vi "Start Measurement.vi"(8 "error in (no error)":errorcluster, 10 "Launch Measurements Message in":refnum<class "Launch Measurements Message.lvclass">, 11 "Controller in":refnum<class "Controller.lvclass">) -> (0 "error out":errorcluster, 3 "Controller out":refnum<class "Controller.lvclass">)   [LabVIEW 2016, in "Controller Actor.lvlib" / "Controller.lvclass"]
uses:
  <userlib>/Common Components/Controller/Controller.lvclass
  C:/Program Files (x86)/National Instruments/LabVIEW 2016/vi.lib/ActorFramework/Actor/Actor.lvclass
  <userlib>/Common Components/Controller/Messages/Launch Measurements Message/Launch Measurements Message.lvclass
  <userlib>/Common Components/Controller/Messages/Launch Measurements Message/Launch Measurements Message.lvclass/Launch Measurements Message.ctl
  <userlib>/Common Components/Function Actor/Function.lvclass/Function.ctl
  <vilib>/ActorFramework/Actor/Actor.lvclass/Actor.ctl
  <vilib>/ActorFramework/Message Enqueuer/Message Enqueuer.lvclass/Message Enqueuer.ctl
  <userlib>/Common Components/Function Actor/Accessors/Write Time Measurement Requested.vi
  <userlib>/Common Components/Function Actor/Write GUID.vi
  <userlib>/Common Components/Controller/Messages/Launch Measurements Message/Read Measurement Name.vi
  <userlib>/Common Components/Controller/Messages/Launch Measurements Message/Read Device Names.vi
  <userlib>/Common Components/Controller/Messages/Launch Measurements Message/Read Show FP_.vi
  <userlib>/Common Components/Controller/Messages/Launch Measurements Message/Read Time Measurement Requested 2.vi
  <userlib>/Common Components/Controller/Messages/Launch Measurements Message/Read GUID.vi
  <vilib>/ActorFramework/Message Enqueuer/Init from Existing Queue.vi
  <userlib>/Common Components/Function Actor/Function.lvclass
  <userlib>/Common Components/Function Actor/Properties/Write Array of Hardware 2.vi
  <userlib>/Common Components/Function Actor/Properties/Write Show UI While Running 2.vi
  <vilib>/ActorFramework/Message Enqueuer/Message Enqueuer.lvclass
  <vilib>/ActorFramework/Actor/Actor.lvclass
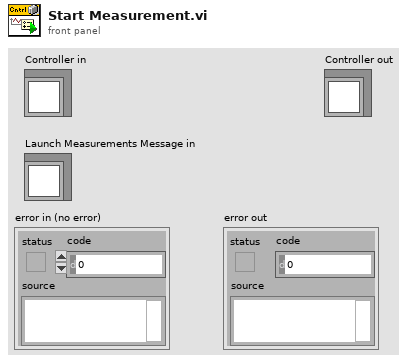
[diagram p1: front panel]
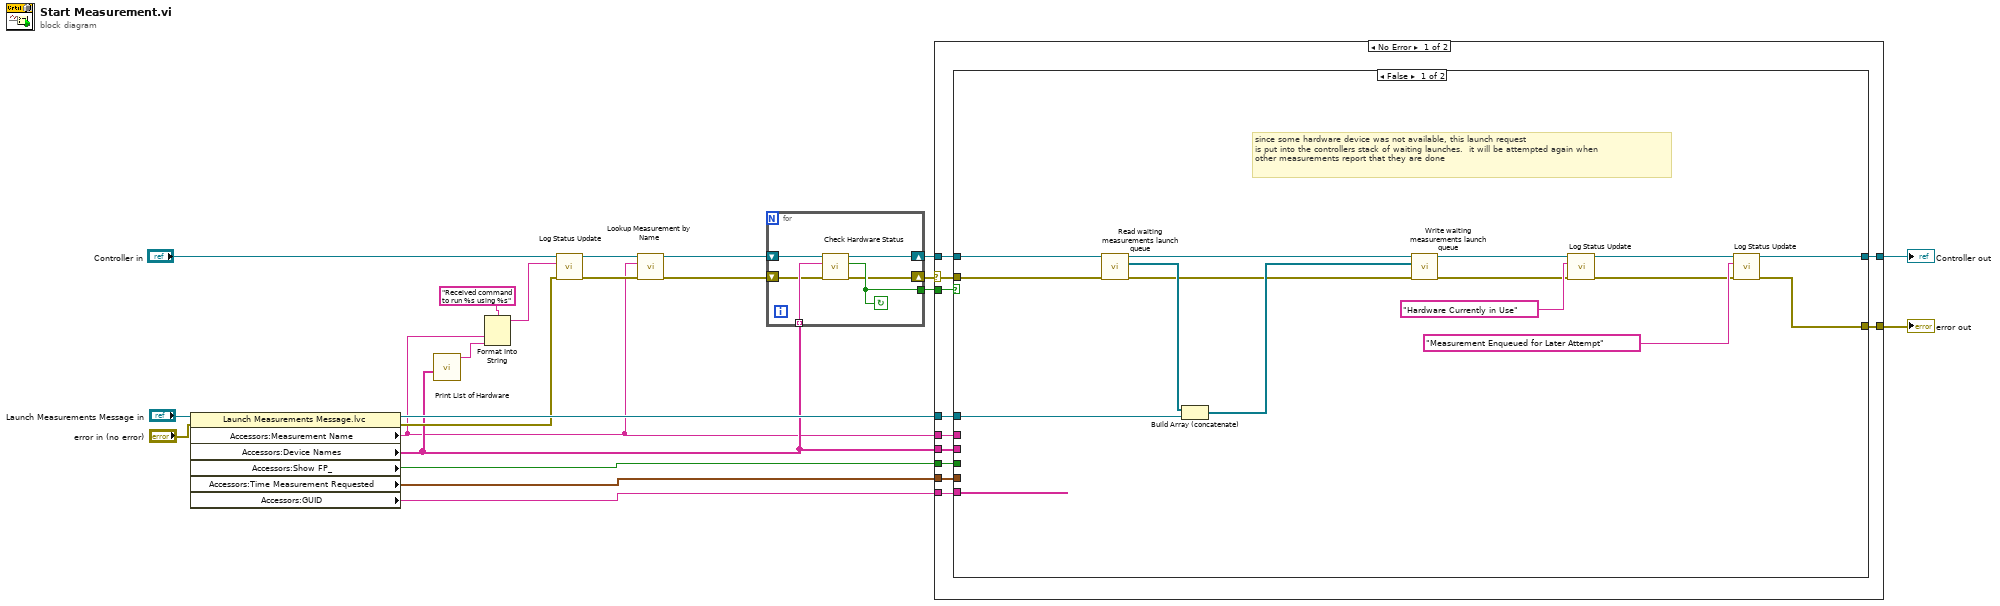
[diagram p0: block diagram]
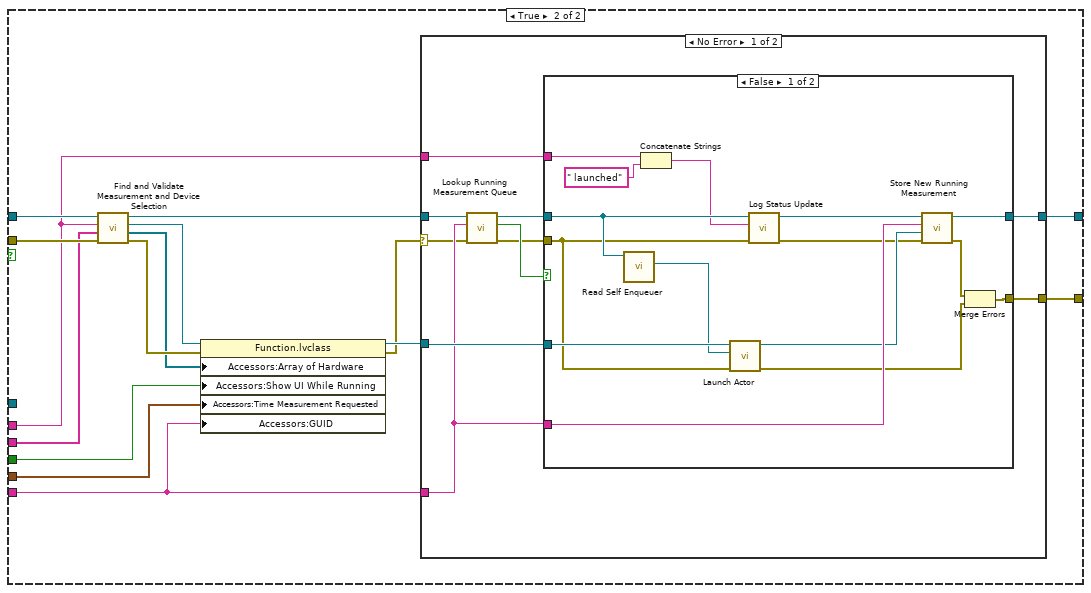
[diagram p2: hidden frame]
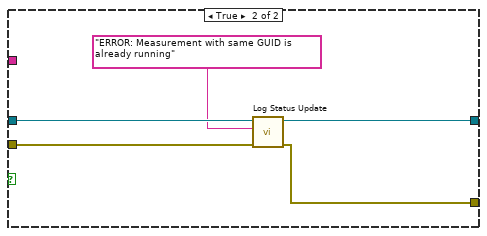
[diagram p3: hidden frame]
diagram:
  n1 = property class="Launch Measurements Message.lvc"(reference="Launch Measurements Message in", error in="error in (no error)") -> (reference out=w12:refnum<class "Launch Measurements Message.lvclass">, error out=w7:errorcluster, "Accessors:Measurement Name"=w1:string, "Accessors:Device Names"=w6:string[], "Accessors:Show FP_"=w9:bool, "Accessors:Time Measurement Requested"=w8:timestamp, "Accessors:GUID"=w11:string)
  n2 = call <userlib>:"Print List of Hardware.vi"("Device Names"=w6) -> ("String"=w21:string)  [unwired: 10 in]
  n3 = Format Into String(format string="Received command to run %s using %s", w1, w21) -> (resulting string=w20:string)  [unwired: 2 in, 1 out]
  n4 = call-dynamic "Log Status Update.vi"("error in (no error)"=w7, "String"=w20, "Controller in"="Controller in") -> ("error out"=w4:errorcluster, "Controller out"=w5:refnum<class "Controller.lvclass">)  [unwired: 7 in]
  n5 = call <userlib>:"Lookup Measurement by Name.vi"("error in (no error)"=w4, "Measurement Name"=w1, "Controller in"=w5) -> ("error out"=w3:errorcluster, "Controller out"=w2:refnum<class "Controller.lvclass">)  [unwired: 5 in, 2 out]
  n6 = for {
    shift-right: [w27] -> w17
    shift-left: w2 -> [w28]
    tunnel: w6 -> [w26] mode=indexing
    tunnel: [w25] -> w18
    shift-right: [w24] -> w16
    shift-left: w3 -> [w23]
    stop <- w25 continue-if-true
    n7 = call <userlib>:"Check Hardware Status.vi"("error in (no error)"=w23, "Device Name"=w26, "Controller in"=w28) -> ("error out"=w24:errorcluster, "Available?"=w25:bool, "Controller out"=w27:refnum<class "Controller.lvclass">)  [unwired: 6 in]
  }
  n8 = case shown="No Error" w16 {
    selector: w16 -> [w33 w103]
    tunnel: w18 -> [w39 _]
    tunnel: w17 -> [w38 w102]
    tunnel: [w37 w102] -> w14
    tunnel: w11 -> [w36 _]
    tunnel: [w35 w103] -> w13
    tunnel: w12 -> [w34 _]
    tunnel: w9 -> [w32 _]
    tunnel: w8 -> [w31 _]
    tunnel: w1 -> [w30 _]
    tunnel: w6 -> [w29 _]
    frame No Error {
      n9 = case shown="False" w39 {
        tunnel: [w41 w69] -> w37
        tunnel: w38 -> [w52 w67]
        tunnel: w33 -> [w50 w66]
        tunnel: [w42 w65] -> w35
        tunnel: w36 -> [_ w57]
        tunnel: w34 -> [w40 _]
        tunnel: w32 -> [_ w55]
        tunnel: w31 -> [_ w56]
        tunnel: w30 -> [_ w58]
        tunnel: w29 -> [_ w59]
        frame False {
          # "since some hardware device was not available, this launch request\nis put into the controllers stack of waiting launches.  it will be attempted again when\nother measurements report that they are done"
          n10 = call <userlib>:"Read waiting measurements launch queue.vi"("error in (no error)"=w50, "Controller in"=w52) -> ("error out"=w49:errorcluster, "stack of waiting msmt requests"=w54:refnum<class "Launch Measurements Message.lvclass">[], "Controller out"=w53:refnum<class "Controller.lvclass">)  [unwired: 7 in]
          n11 = Build Array (concatenate)(w54, w40) -> (w51:refnum<class "Launch Measurements Message.lvclass">[])
          n12 = call <userlib>:"Write waiting measurements launch queue.vi"("error in (no error)"=w49, "stack of waiting msmt requests"=w51, "Controller in"=w53) -> ("error out"=w44:errorcluster, "Controller out"=w45:refnum<class "Controller.lvclass">)  [unwired: 7 in]
          n13 = call-dynamic "Log Status Update.vi"("error in (no error)"=w44, "String"="Hardware Currently in Use", "Controller in"=w45) -> ("error out"=w43:errorcluster, "Controller out"=w46:refnum<class "Controller.lvclass">)  [unwired: 7 in]
          n14 = call-dynamic "Log Status Update.vi"("error in (no error)"=w43, "String"="Measurement Enqueued for Later Attempt", "Controller in"=w46) -> ("error out"=w42:errorcluster, "Controller out"=w41:refnum<class "Controller.lvclass">)  [unwired: 7 in]
        }
        frame True {
          n15 = call <userlib>:"Find and Validate Measurement and Device Selection.vi"("error in (no error)"=w66, "Device Names"=w59, "Measurement Name"=w58, "Controller in"=w67) -> ("error out"=w63:errorcluster, "Hardware Objects"=w62:refnum<class "Hardware.lvclass">[], "Measurement out"=w61:refnum<class "Function.lvclass">, "Controller out"=w64:refnum<class "Controller.lvclass">)  [unwired: 4 in]
          n16 = property class="Function.lvclass"(reference=w61, error in=w63, "Accessors:Array of Hardware"=w62, "Accessors:Show UI While Running"=w55, "Accessors:Time Measurement Requested"=w56, "Accessors:GUID"=w57) -> (reference out=w68:refnum<class "Function.lvclass">, error out=w60:errorcluster)
          n17 = case shown="No Error" w60 {
            selector: w60 -> [w71 w101]
            tunnel: [w79 w100] -> w69
            tunnel: w68 -> [w75 _]
            tunnel: w64 -> [w74 w100]
            tunnel: w57 -> [w73 _]
            tunnel: [w72 w101] -> w65
            tunnel: w58 -> [w70 _]
            frame No Error {
              n18 = call <userlib>:"Lookup Running Measurement Queue.vi"("error in (no error)"=w71, "Measurement Name.Harware()"=w73, "Controller in"=w74) -> ("error out"=w76:errorcluster, "Found?"=w77:bool, "Controller out"=w78:refnum<class "Controller.lvclass">)  [unwired: 5 in, 1 out]
              n19 = case shown="False" w77 {
                tunnel: [w94 w98] -> w79
                tunnel: w75 -> [w93 _]
                tunnel: w73 -> [w92 _]
                tunnel: w78 -> [w90 w99]
                tunnel: w76 -> [w84 w96]
                tunnel: [w81 w95] -> w72
                tunnel: w70 -> [w80 _]
                frame False {
                  n20 = call <vilib>:"Read Self Enqueuer.vi"("Actor"=w90) -> ("Self Enqueuer"=w89:refnum<class "Message Enqueuer.lvclass">)  [unwired: 10 in]
                  n21 = Concatenate Strings(w80, " launched" ("string")) -> (w86:string)
                  n22 = call <vilib>:"Launch Actor.vi"("error in (no error)"=w84, "Actor-to-Caller Enqueuer"=w89, "Actor"=w93) -> ("error out"=w82:errorcluster, "Caller-To-Actor Enqueuer"=w88:refnum<class "Message Enqueuer.lvclass">)  [unwired: 7 in]
                  n23 = call-dynamic "Log Status Update.vi"("error in (no error)"=w84, "String"=w86, "Controller in"=w90) -> ("error out"=w85:errorcluster, "Controller out"=w87:refnum<class "Controller.lvclass">)  [unwired: 7 in]
                  n24 = call <userlib>:"Store New Running Measurement.vi"("error in (no error)"=w85, "Caller-To-Actor Enqueuer"=w88, "name"=w92, "Controller in"=w87) -> ("error out"=w83:errorcluster, "Controller out"=w94:refnum<class "Controller.lvclass">)  [unwired: 6 in]
                  n25 = Merge Errors(w83, w82) -> (w81:errorcluster)
                }
                frame True {
                  n26 = call-dynamic "Log Status Update.vi"("error in (no error)"=w96, "String"="ERROR: Measurement with same GUID is already running", "Controller in"=w99) -> ("error out"=w95:errorcluster, "Controller out"=w98:refnum<class "Controller.lvclass">)  [unwired: 7 in]
                }
              }
            }
            frame Error {
            }
          }
        }
      }
    }
    frame Error {
    }
  }
  "error out" <- w13
  "Controller out" <- w14
